vi "Get spacing value for control type.vi"(8 "error in":errorcluster, 11 "control reference in":refnum<vi>) -> (0 "error out":errorcluster, 2 "Spacing value":u32, 3 "control reference out":refnum<vi>)   [LabVIEW 2020, in "verticalDistribution.lvlib"]
uses:
  <vilib>/Utility/vertDist/verticalDistribution.lvlib
  <vilib>/Utility/vertDist/SectionLabel.ctl
  <vilib>/Utility/vertDist/FirstSectionLabel.ctl
panel:
  out "First Section":T1="Sample First Section"
  out "General Section":T2="Sample Section"
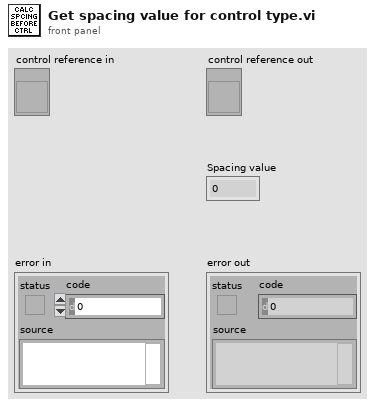
[diagram p1: front panel]
types:
  T1 = typedef "verticalDistribution.lvlib/FirstSectionLabel.ctl" = string
  T2 = typedef "verticalDistribution.lvlib/SectionLabel.ctl" = string
  T3 = enum32{"not a typedef", "typedef", "strict typedef", "class private data"}
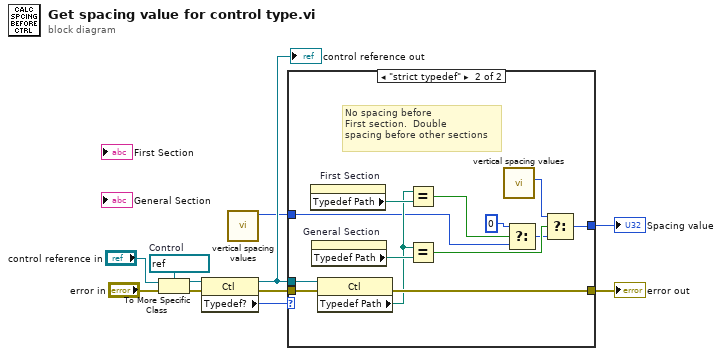
[diagram p0: block diagram]
diagram:
  w7 = refnum<vi> refnum  # Control
  n1 = To More Specific Class(target class=w7, reference="control reference in", error in="error in") -> (specific class reference=w6:refnum<vi>, error out=w10:errorcluster)
  n2 = property class="Ctl"(reference=w6, error in=w10) -> (reference out=w4:refnum<vi>, error out=w9:errorcluster, "Typedef?"=w5:T3)
  "control reference out" <- w4
  n3 = call <vilib>:"vertical spacing values.vi"() -> ("Control spacing"=w3:u32)  [unwired: 3 out]
  n4 = case shown="\"strict typedef\"" w5 {
    tunnel: [w12 w24] -> w2
    tunnel: w4 -> [_ w22]
    tunnel: w3 -> [w12 w14]
    tunnel: w9 -> [w13 w26]
    tunnel: [w13 w25] -> w8
    frame Default {
    }
    frame "strict typedef" {
      # "No spacing before\nFirst section.  Double\nspacing before other sections"
      n5 = property on="First Section" class="Str (strict)"() -> ("Typedef Path"=w19:path)  [unwired: 2 in, 2 out]
      n6 = property on="General Section" class="Str (strict)"() -> ("Typedef Path"=w21:path)  [unwired: 2 in, 2 out]
      n7 = property class="Ctl"(reference=w22, error in=w26) -> (error out=w25:errorcluster, "Typedef Path"=w18:path)  [unwired: 1 out]
      n8 = Equal?(x=w18, y=w19) -> (x = y?=w16:bool)
      n9 = Equal?(x=w18, y=w21) -> (x = y?=w20:bool)
      n10 = call <vilib>:"vertical spacing values.vi"() -> ("Section spacing"=w23:u32)  [unwired: 3 out]
      n11 = Select(t=0, s=w16, f=w14) -> (s? t:f=w17:u32)
      n12 = Select(t=w23, s=w20, f=w17) -> (s? t:f=w24:u32)
    }
  }
  "Spacing value" <- w2
  "error out" <- w8
